vi "PID.vi"(0 "当前值":dbl, 1 "kp":dbl, 2 "ki":dbl, 3 "kd":dbl, 4 "目标值":dbl) -> (5 "输出值":dbl)   [LabVIEW 2022 SP3]
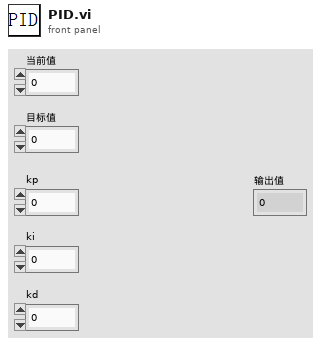
[diagram p1: front panel]
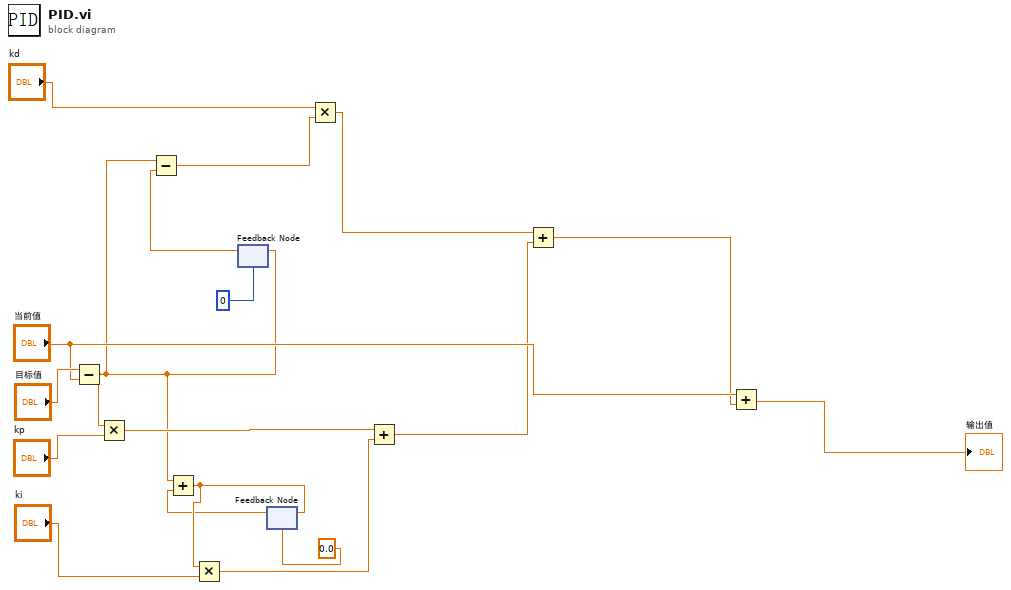
[diagram p0: block diagram]
diagram:
  n1 = Subtract(x="目标值", y="当前值") -> (x-y=w2:dbl)
  n2 = Multiply(x=w2, y="kp") -> (x*y=w11:dbl)
  n3 = feedback-in #1(w2) -> ()
  n4 = feedback #1(0) -> (w8:dbl)
  n5 = Subtract(x=w2, y=w8) -> (x-y=w6:dbl)
  n6 = feedback #2(0.0) -> (w14:dbl)
  n7 = Add(x=w2, y=w14) -> (x+y=w17:dbl)
  n8 = Multiply(x=w17, y="ki") -> (x*y=w15:dbl)
  n9 = feedback-in #2(w17) -> ()
  n10 = Multiply(x="kd", y=w6) -> (x*y=w5:dbl)
  n11 = Add(x=w11, y=w15) -> (x+y=w4:dbl)
  n12 = Add(x=w5, y=w4) -> (x+y=w3:dbl)
  n13 = Add(x="当前值", y=w3) -> (x+y=→"输出值":dbl)
